vi "test SeqFileParam parsing.vi"() -> ()   [LabVIEW 2017]
uses:
  LV_Source/Subsystems/Sequencer/DataTypes/SeqFileParameters--cluster.ctl
  LV_Source/Subsystems/Sequencer/DataTypes/SeqFileParam_PosMode--enum.ctl
  LV_Source/Subsystems/Sequencer/DataTypes/SeqFileParam_OscMode--enum.ctl
  LV_Source/Subsystems/Sequencer/Sequencer.lvclass
panel:
  out "text lines out":string[](array[string])
  out "SeqFileParams":T1
  out "error out":errorcluster
  in  "SeqFile":path
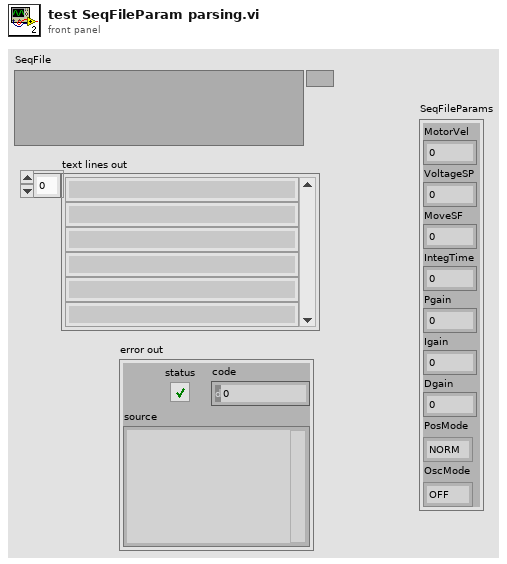
[diagram p1: front panel]
types:
  T1 = typedef "Sequencer.lvclass/SeqFileParameters--cluster.ctl" = cluster{"MotorVel":dbl, "VoltageSP":dbl, "MoveSF":dbl, "IntegTime":dbl, "Pgain":dbl, "Igain":dbl, "Dgain":dbl, "PosMode":T2, "OscMode":T3}
  T2 = typedef "Sequencer.lvclass/SeqFileParam_PosMode--enum.ctl" = enum16{"NORM", "ABS"}
  T3 = typedef "Sequencer.lvclass/SeqFileParam_OscMode--enum.ctl" = enum16{"OFF", "ON"}
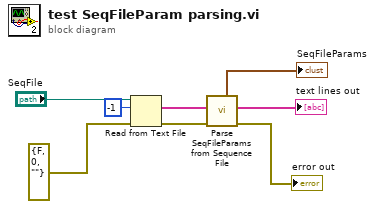
[diagram p0: block diagram]
diagram:
  n1 = Read from Text File(file (use dialog)="SeqFile", count=-1, error in=errorcluster {"status"=FALSE, "code"=0, "source"=""}) -> (text=w7:string[], error out=w5:errorcluster)  [unwired: 1 in, 2 out]
  n2 = call "Parse SeqFileParams from Sequence File.vi"("error in (no error)"=w5, "text lines in"=w7) -> ("error out"=→"error out":errorcluster, "text lines out"=→"text lines out":string[], "SeqFileParams"=→"SeqFileParams":T1)  [unwired: 7 in]
